vi "CV_config_LCR.vi"(0 "Input parameters":T1={"Measurement type"=enum."Debug", "Sensor type"=enum."HPK_8in_271ch", "Identifier"="test.txt", "Open after execution?"=FALSE, "Plot after execution?"=FALSE, "Display channel"=0, "Voltage Delay (s)"=0.5, "Switch Delay (s)"=0.01, "VISA resource name source"="", "VISA resource name DMM"="", "VISA resource name LCR"="", "Compliance  Level (A)"=10.0, "Voltage Limit (V)"=1000.0, "Data storage location"="", "Scan voltages"="", "Use source as DMM?"=FALSE, "LCR signal frequenzy (Hz)"=10.0, "DMM device"=enum."Keithley2001", "Sampling number"=1, "Use env. sensors on"=enum."Sensirion sht1x/7x", "Switchboard Handle"=0, "Use Switchboard"=FALSE, "LCR signal voltage (V)"=10000.0, "Repeat"=1, "Scan voltages IV"="", "Scan voltages CV"="", "Hex pad numbers?"=FALSE, "Set measurement type"=enum."Debug", "Custom pad scan"="", "IV voltage Delay (s)"=0.5, "CV voltage Delay (s)"=0.5, "Needle measurement?"=FALSE, "Comments"="test.txt", "LCR signal frequenzy (kHz)"=10.0, "Compliance  Level (uA)"=10.0, "Open Correction Array"=array2304x3[6912 elements], "Current set voltage"=0.0, "Last set voltage"=0.0, "Current channel"=0, "Last OpenCorrection index"=-1, "Total curr/vltg every x steps"=10, "Current channel iteration"=0, "No CV corrections"=FALSE, "Mapfile"="", "Corrfile"="", "IV voltage file"=path "", "CV voltage file"=path "", "IV Switch Delay (s)"=0.01, "CV Switch Delay (s)"=0.01, "Invert polarity"=FALSE, "Set debug dirs"=FALSE, "Is n on p"=FALSE, "Source interlock?"=TRUE, "Voltage file used?"=FALSE, "Pad mask"="", "Mask pad above (uA)"=1.0, "LCR device"=enum."LCR_E4980", "Source device"=enum."Source_2410", "HexPlot binary path"="", "PadReductionFactor"=1.0, "Temperature degC"="", "Fluence [neq]"="", "Annealing [min]"=""} {"CV Switch Delay (s)" format="%#_13g"; "IV Switch Delay (s)" format="%#_13g"; "Last set voltage" format="%#_13g"; "Current set voltage" format="%#_13g"; "CV voltage Delay (s)" format="%#_13g"; "IV voltage Delay (s)" format="%#_13g"; "Voltage Limit (V)" format="%#_13g"; "Voltage Delay (s)" format="%#_13g"; "Switch Delay (s)" format="%#_13g"}, 11 "error in (no error)":errorcluster) -> (4 "VISA resource name out":refnum<visa-resource-name>, 15 "error out":errorcluster)   [LabVIEW 2020]
doc: "Sets the configuration for the LCR meter."
uses:
  input_params.ctl
  <instrlib>/Agilent E4980/Agilent E4980.lvlib
  <instrlib>/Agilent 4263X/Agilent 4263X.lvlib
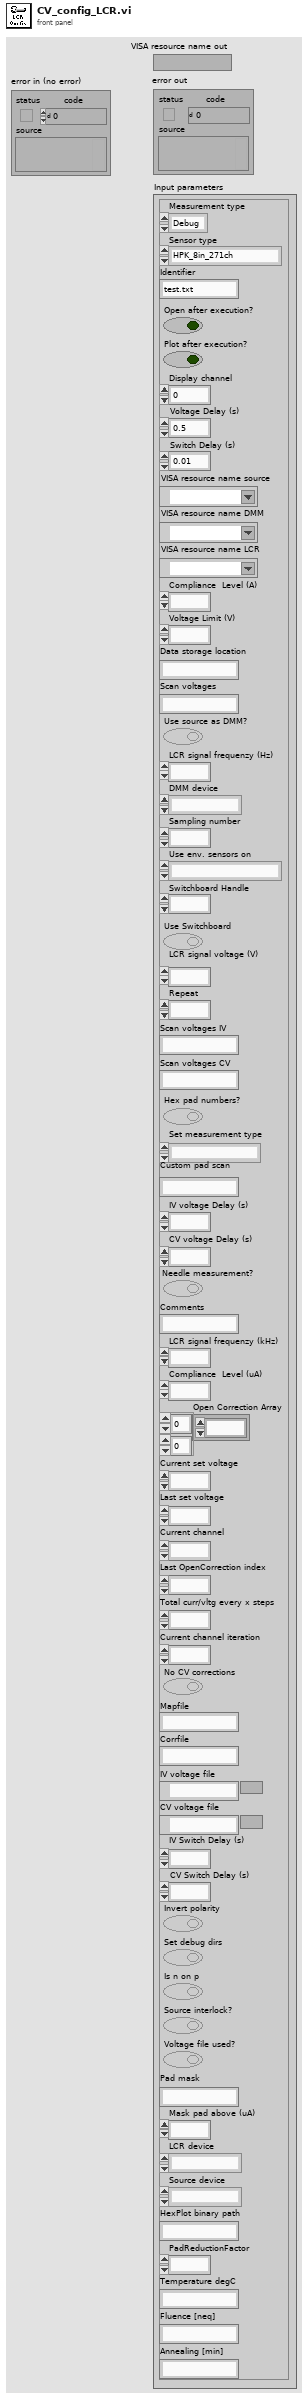
[diagram p1: front panel]
types:
  T1 = typedef "input_params.ctl" = cluster{"Measurement type":enum16{"IV", "CV", "Debug", "Test_contact"}, "Sensor type":enum16{"HPK_6in_135ch", "HPK_8in_271ch", "IFX_8in_256ch", "Diode", "HPK_6in_239ch", "Full_Matrix", "HPK_8in_271ch_full", "LumiCal", "HPK_8in_444ch", "HPK_8in_198ch_2019", "HPK_8in_MGW_LD_full", "HPK_8in_MGW_LD_a_type_top", "HPK_8in_MGW_LD_a_type_bottom", "HPK_8in_MGW_LD_b_type_left", "HPK_8in_MGW_LD_b_type_right", "HPK_8in_MGW_LD_c_type_left", "HPK_8in_MGW_LD_c_type_right", "HPK_8in_MGW_HD_full", "HPK_8in_MGW_HD_a_type_top", "HPK_8in_MGW_HD_a_type_bottom", "HPK_8in_MGW_HD_b_type_left", "HPK_8in_MGW_HD_b_type_right", "HPK_8in_MGW_HD_c_type_left", "HPK_8in_MGW_HD_c_type_right", "CALICE_6in_256ch"}, "Identifier":string, "Open after execution?":bool, "Plot after execution?":bool, "Display channel":i32, "Voltage Delay (s)":dbl, "Switch Delay (s)":dbl, "VISA resource name source":refnum<visa-resource-name>, "VISA resource name DMM":refnum<visa-resource-name>, "VISA resource name LCR":refnum<visa-resource-name>, "Compliance  Level (A)":dbl, "Voltage Limit (V)":dbl, "Data storage location":string, "Scan voltages":string, "Use source as DMM?":bool, "LCR signal frequenzy (Hz)":dbl, "DMM device":enum16{"Keithley2001", "Keithley2450", "Keithley2410", "Keithley6485", "Keithley6487", "Keithley6517"}, "Sampling number":i32, "Use env. sensors on":enum16{"Sensirion sht1x/7x", "Switch Matrix", "Probecard"}, "Switchboard Handle":u32, "Use Switchboard":bool, "LCR signal voltage (V)":dbl, "Repeat":i32, "Scan voltages IV":string, "Scan voltages CV":string, "Hex pad numbers?":bool, "Set measurement type":enum16{"IV", "CV", "Debug", "Test_contact", "IV+CV"}, "Custom pad scan":string, "IV voltage Delay (s)":dbl, "CV voltage Delay (s)":dbl, "Needle measurement?":bool, "Comments":string, "LCR signal frequenzy (kHz)":dbl, "Compliance  Level (uA)":dbl, "Open Correction Array":dbl[][], "Current set voltage":dbl, "Last set voltage":dbl, "Current channel":i32, "Last OpenCorrection index":i32, "Total curr/vltg every x steps":i32, "Current channel iteration":i32, "No CV corrections":bool, "Mapfile":string, "Corrfile":string, "IV voltage file":path, "CV voltage file":path, "IV Switch Delay (s)":dbl, "CV Switch Delay (s)":dbl, "Invert polarity":bool, "Set debug dirs":bool, "Is n on p":bool, "Source interlock?":bool, "Voltage file used?":bool, "Pad mask":string, "Mask pad above (uA)":dbl, "LCR device":enum16{"LCR_E4980", "AGILENT_4263X"}, "Source device":enum16{"Source_2410", "Source_6487", "Source_2470"}, "HexPlot binary path":string, "PadReductionFactor":dbl, "Temperature degC":string, "Fluence [neq]":string, "Annealing [min]":string}
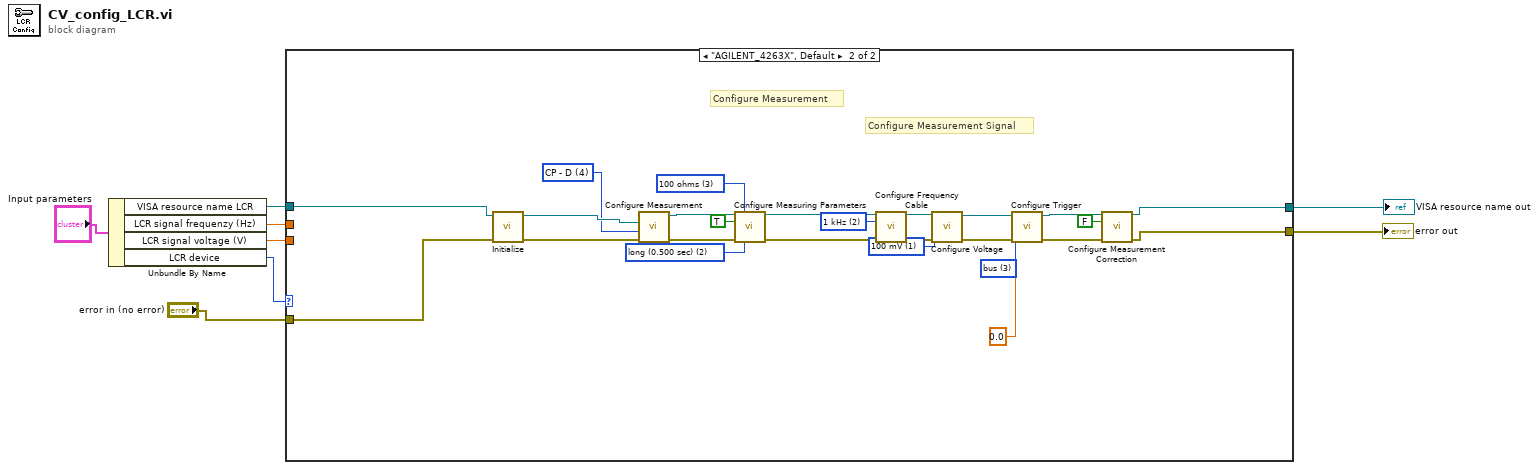
[diagram p0: block diagram]
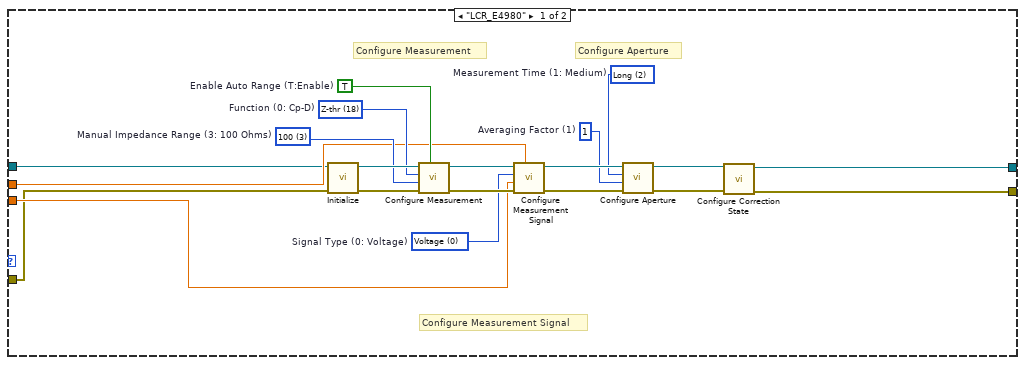
[diagram p2: hidden frame]
diagram:
  n1 = Unbundle By Name("Input parameters") -> ("VISA resource name LCR"=w2:refnum<visa-resource-name>, "LCR signal frequenzy (Hz)"=w6:dbl, "LCR signal voltage (V)"=w7:dbl, "LCR device"=w5:enum16{"LCR_E4980", "AGILENT_4263X"})
  n2 = case shown="\"AGILENT_4263X\", Default" w5 {
    tunnel: w7 -> [w14 _]
    tunnel: w6 -> [w13 _]
    tunnel: [w12 w43] -> w4
    tunnel: [w11 w42] -> w3
    tunnel: w2 -> [w10 w53]
    tunnel: "error in (no error)" -> [w9 w52]
    frame "LCR_E4980" {
      w18 = u16 2 items=["Short", "Medium", "Long"]  # Measurement Time (1: Medium)
      w17 = 1  # Averaging Factor (1)
      w19 = u16 0 items=["Voltage", "Current"]  # Signal Type (0: Voltage)
      w20 = 3 items=["100m", "1", "10", "100", "300", "1K", "3K", "10K", "30K", "100K"]  # Manual Impedance Range (3: 100 Ohms)
      w21 = u16 18 items=["Cp-D", "Cp-Q", "Cp-G", "Cp-Rp", "Cs-D", "Cs-Q", "Cs-Rs", "Lp-D", "Lp-Q", "Lp-G", "Lp-Rp", "Lp-Rdc", "Ls-D", "Ls-Q", "Ls-Rs", "Ls-Rdc", "R-X", "Z-thd", "Z-thr", "G-B", "Y-thd", "Y-thr", "Vdc-Idc"]  # Function (0: Cp-D)
      w22 = TRUE  # Enable Auto Range (T:Enable)
      # "Configure Aperture"
      # "Configure Measurement Signal"
      # "Configure Measurement"
      n3 = call <instrlib>:"Initialize.vi"("error in (no error)"=w9, "VISA resource name"=w10) -> ("error out"=w27:errorcluster, "VISA resource name out"=w28:refnum<visa-resource-name>)  [unwired: 8 in]
      n4 = call <instrlib>:"Configure Measurement.vi"("Enable Auto Range (T:Enable)"=w22, "error in (no error)"=w27, "Manual Impedance Range (3: 100 Ohms)"=w20, "Function (0: Cp-D)"=w21, "VISA resource name"=w28) -> ("error out"=w25:errorcluster, "VISA resource name out"=w26:refnum<visa-resource-name>)  [unwired: 5 in]
      n5 = call <instrlib>:"Configure Measurement Signal.vi"("Signal Frequency (1000 Hz)"=w13, "error in (no error)"=w25, "Signal Level (1.0 V)"=w14, "Signal Type (0: Voltage)"=w19, "VISA resource name"=w26) -> ("error out"=w23:errorcluster, "VISA resource name out"=w24:refnum<visa-resource-name>)  [unwired: 5 in]
      n6 = call <instrlib>:"Configure Aperture.vi"("error in (no error)"=w23, "Averaging Factor (1)"=w17, "Measurement Time (1: Medium)"=w18, "VISA resource name"=w24) -> ("error out"=w16:errorcluster, "VISA resource name out"=w15:refnum<visa-resource-name>)  [unwired: 6 in]
      n7 = call <instrlib>:"Configure Correction State.vi"("error in (no error)"=w16, "VISA resource name"=w15) -> ("error out"=w11:errorcluster, "VISA resource name out"=w12:refnum<visa-resource-name>)  [unwired: 8 in]
    }
    frame "AGILENT_4263X", Default {
      w29 = u16 1 items=["50 mV", "100 mV", "250 mV", "500 mV", "1 V", "20 mV"] ("level (50mV)")
      w30 = u16 2 items=["100 Hz", "120 Hz", "1 kHz", "10 kHz", "20 kHz (option 002 ONLY)", "100 kHz"] ("frequency (100 Hz)")
      w32 = u16 2 items=["short (0.025 sec)", "medium (0.065 sec)", "long (0.500 sec)"] ("aperture (short:0)")
      w34 = u16 3 items=["0.1 ohms", "1 ohm", "10 ohms", "100 ohms", "1k ohms", "10k ohms", "100k ohms", "1M ohms"] ("range (1 ohm:1)")
      w35 = u16 4 items=["Z - Angle", "R - X", "Y - Angle", "G - B", "CP - D", "CP - Q", "CP - G", "CS - D", "CS - Q", "CS - RS", "LP - D", "LP - Q", "LP - G", "LS - D", "LS - Q", "LS - RS", "LS - DCR (option 001 only)", "LP - DCR (option 001 only)", "L2 - N (option 001 only)", "L2 - M (option 001 only)", "L2 - R2 (option 001 only)"] ("function (Z - Angle:0)")
      w41 = u16 3 items=["internal", "external", "manual", "bus"] ("trigger source (int:0)")
      # "Configure Measurement Signal"
      # "Configure Measurement"
      n8 = call <instrlib>:"Initialize.vi"("error in (no error)"=w52, "VISA resource name"=w53) -> ("error out"=w51:errorcluster, "VISA resource name out"=w50:refnum<visa-resource-name>)  [unwired: 8 in]
      n9 = call <instrlib>:"Configure Measurement.vi"("error in (no error)"=w51, "function (Z - Angle:0)"=w35, "VISA resource name"=w50) -> ("error out"=w48:errorcluster, "VISA resource name out"=w49:refnum<visa-resource-name>)  [unwired: 7 in]
      n10 = call <instrlib>:"Configure Measuring Parameters.vi"("VISA resource name"=w49, "range (1 ohm:1)"=w34, "Auto Range (T)"=TRUE, "error in (no error)"=w48, "aperture (short:0)"=w32) -> ("VISA resource name out"=w47:refnum<visa-resource-name>, "error out"=w45:errorcluster)  [unwired: 9 in]
      n11 = call <instrlib>:"Configure Frequency Cable.vi"("VISA resource name"=w47, "frequency (100 Hz)"=w30, "error in (no error)"=w45) -> ("VISA resource name out"=w46:refnum<visa-resource-name>, "error out"=w44:errorcluster)  [unwired: 11 in]
      n12 = call <instrlib>:"Configure Voltage.vi"("VISA resource name"=w46, "level (50mV)"=w29, "error in (no error)"=w44) -> ("VISA resource name out"=w37:refnum<visa-resource-name>, "error out"=w36:errorcluster)  [unwired: 11 in]
      n13 = call <instrlib>:"Configure Trigger.vi"("error in (no error)"=w36, "trigger delay (sec)"=0.0, "trigger source (int:0)"=w41, "VISA resource name"=w37) -> ("error out"=w39:errorcluster, "VISA resource name out"=w38:refnum<visa-resource-name>)  [unwired: 6 in]
      n14 = call <instrlib>:"Configure Measurement Correction.vi"("VISA resource name"=w38, "enable correction (T)"=FALSE, "error in (no error)"=w39) -> ("VISA resource name out"=w43:refnum<visa-resource-name>, "error out"=w42:errorcluster)  [unwired: 11 in]
    }
  }
  "VISA resource name out" <- w4
  "error out" <- w3
